vi "window1.vi"() -> ()   [LabVIEW 2014]
uses:
  FG states.ctl
  child window props.ctl
panel:
  out "Waveform Chart":dbl(graph)
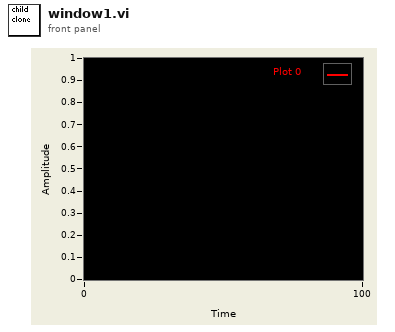
[diagram p1: front panel]
types:
  T1 = typedef "child window props.ctl" = cluster{"WindowTitle":string, "hWnd":u32, "VI Refnum":refnum<vi>}
  T2 = typedef "FG states.ctl" = enum16{"init", "add", "replace", "remove", "read"}
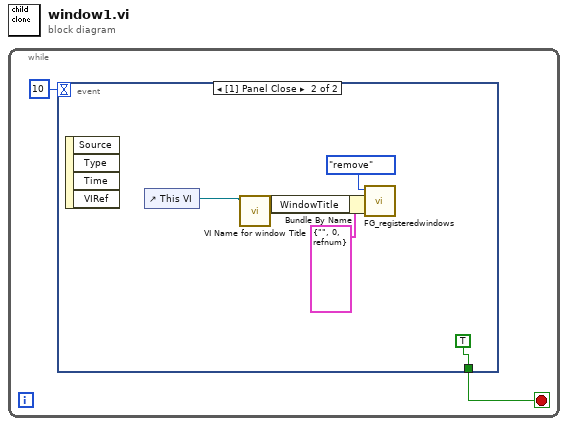
[diagram p0: block diagram]
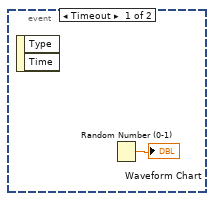
[diagram p2: hidden frame]
diagram:
  n1 = while {
    stop <- w1 stop-if-true
    n2 = event shown="[1] Panel Close" {
      selector: _ -> [_ _]
      dyn-events: _ -> [_ _]
      timeout: 10 -> [_ _]
      tunnel: [_ TRUE] -> w1
      event Timeout {
        n3 = event-data() -> ()  [unwired: 3 out]
        n4 = Random Number (0-1)() -> (number: 0 to 1=→"Waveform Chart":dbl)
      }
      event Panel Close {
        n5 = event-data() -> ()  [unwired: 5 out]
        n6 = control-ref of="This VI"() -> (w5:refnum<vi>)
        n7 = call "VI Name for window Title.vi"("vi reference"=w5) -> ("Vi tiltle"=w4:string)  [unwired: 1 in, 9 out]
        n8 = Bundle By Name(cluster=T1 {"WindowTitle"="", "hWnd"=0, "VI Refnum"=refnum} ("window"), "WindowTitle"=w4) -> (w7:T1)
        n9 = call "FG_registeredwindows.vi"("window"=w7, "action"=FG_states."remove") -> ()  [unwired: 1 in, 9 out]
      }
    }
  }
